vi "Error Cleanup.vi"(8 "error in (no error)":errorcluster, 11 "RS232 to GPIB ConvBox in":refnum<class "RS-xxx to GPIB ConvBox.lvclass">) -> (0 "error out":errorcluster, 3 "RS232 to GPIB ConvBox out":refnum<class "RS-xxx to GPIB ConvBox.lvclass">)   [LabVIEW 2023, in "Protocols.lvlib" / "RS-xxx to GPIB ConvBox.lvclass"]
uses:
  RS-xxx to GPIB ConvBox.lvclass
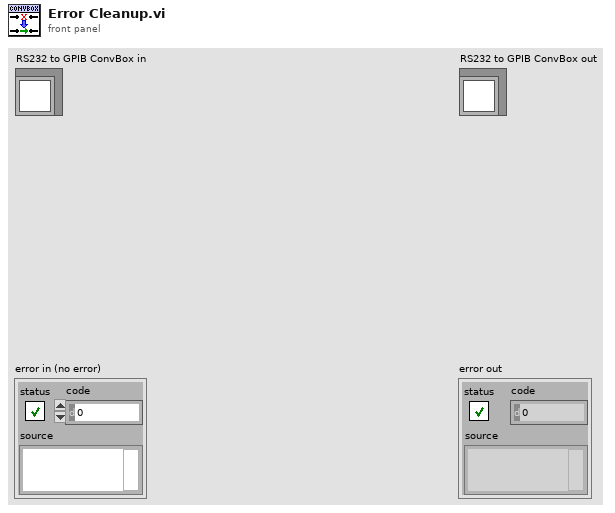
[diagram p1: front panel]
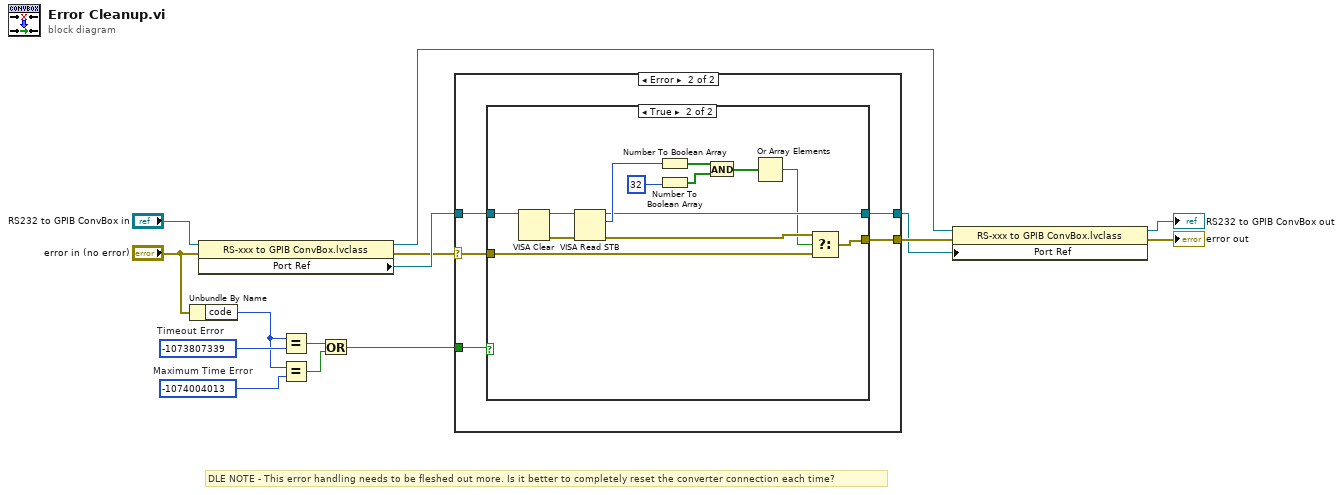
[diagram p0: block diagram]
diagram:
  w10 = -1074004013  # Maximum Time Error
  w15 = -1073807339  # Timeout Error
  # "DLE NOTE - This error handling needs to be fleshed out more. Is it better to completely reset the converter connection each time?"
  n1 = Unbundle By Name("error in (no error)") -> ("code"=w11:i32)
  n2 = property class="RS-xxx to GPIB ConvBox.lvclass"(reference="RS232 to GPIB ConvBox in", error in="error in (no error)") -> (reference out=w5:refnum<class "RS-xxx to GPIB ConvBox.lvclass">, error out=w8:errorcluster, "Port Ref"=w9:refnum<visa-resource-name>)
  n3 = Equal?(x=w11, y=w15) -> (x = y?=w14:bool)
  n4 = Equal?(x=w11, y=w10) -> (x = y?=w12:bool)
  n5 = Or(x=w14, y=w12) -> (x .or. y?=w13:bool)
  n6 = case shown="Error" w8 {
    selector: w8 -> [w16 w20]
    tunnel: w9 -> [w17 w22]
    tunnel: [w17 w21] -> w6
    tunnel: [w16 w19] -> w7
    tunnel: w13 -> [_ w18]
    frame No Error {
    }
    frame Error {
      n7 = case shown="True" w18 {
        tunnel: w22 -> [w24 w34]
        tunnel: [w24 w29] -> w21
        tunnel: w20 -> [w23 w26]
        tunnel: [w23 w27] -> w19
        frame False {
        }
        frame True {
          n8 = VISA Clear(VISA resource name=w34) -> (VISA resource name out=w36:refnum<visa-resource-name>, error out=w37:errorcluster)  [unwired: 1 in]
          n9 = VISA Read STB(8:w37, 11:w36) -> (0:w28:errorcluster, 2:w33:u16, 3:w29:refnum<visa-resource-name>)
          n10 = Number To Boolean Array(number=w33) -> (Boolean array=w32:bool[])
          n11 = Number To Boolean Array(number=u32 32 ("l")) -> (Boolean array=w31:bool[])
          n12 = And(x=w32, y=w31) -> (x .and. y?=w30:bool[])
          n13 = Or Array Elements(Boolean array=w30) -> (logical OR=w25:bool)
          n14 = Select(t=w28, s=w25, f=w26) -> (s? t:f=w27:errorcluster)
        }
      }
    }
  }
  n15 = property class="RS-xxx to GPIB ConvBox.lvclass"(reference=w5, error in=w7, "Port Ref"=w6) -> (reference out=→"RS232 to GPIB ConvBox out":refnum<class "RS-xxx to GPIB ConvBox.lvclass">, error out=→"error out":errorcluster)
